vi "Benchmark VIReg(SubVI).vi"(11 "#Tags":i32) -> (0 "Values":dbl[](array[numeric]), 1 "Read Time":dbl, 2 "Write Time":dbl, 3 "Creation Time":dbl)   [LabVIEW 2019]
uses:
  <vilib>/GPower/VIRegister/Library/Typedefs/RegisterType.ctl
  <vilib>/GPower/VIRegister/Library/Convert/ToDBL.vi
  <vilib>/GPower/VIRegister/Library/QManager/CreateRegister.vi
  <vilib>/GPower/VIRegister/Library/SubVIs/FindRegisterData.vi
  <vilib>/GPower/VIRegister/Library/SubVIs/WriteSub.vi
  <vilib>/GPower/VIRegister/Library/SubVIs/ReadSub.vi
  <vilib>/GPower/Error/Library/IsError.vi
  <vilib>/GPower/VIRegister/Library/QManager/ReleaseAll.vi
  <vilib>/GPower/VIRegister/Library/QManager/QManagerAction.vi
  <vilib>/GPower/VIRegister/Library/QManager/GetRegisterData.vi
  <vilib>/GPower/Error/Library/SetError.vi
  <vilib>/GPower/Error/Library/FilterCodes.vi
  <vilib>/GPower/Error/Library/Filter/FilterMulti.vi
  <vilib>/GPower/Error/Library/ErrorType.vi
  <vilib>/GPower/Error/Library/SplitAppended.vi
  <vilib>/GPower/Error/Library/SubVIs/ExplanationToError.vi
  <vilib>/dlg_ctls.llb/Space Constant.vi
  <vilib>/GPower/VIRegister/Library/QManager/GetQName.vi
  <vilib>/GPower/VIRegister/Library/QManager/StartQManager.vi
  <vilib>/Utility/error.llb/Trim Whitespace.vi
  <vilib>/Utility/error.llb/Error Code Database.vi
  <vilib>/GPower/Error/Library/SubVIs/SetStatus.vi
  <vilib>/GPower/Error/Library/AppendErrors.vi
  <vilib>/GPower/Error/Library/Append/AppendSingle.vi
  <vilib>/GPower/VIRegister/VIRegister.lvlib
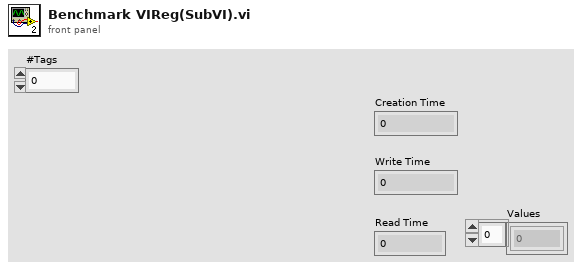
[diagram p1: front panel]
types:
  T1 = typedef "VIRegister.lvlib/RegisterType.ctl" = enum16{"Circular buffer", "FIFO buffer", "LIFO buffer", "Register"}
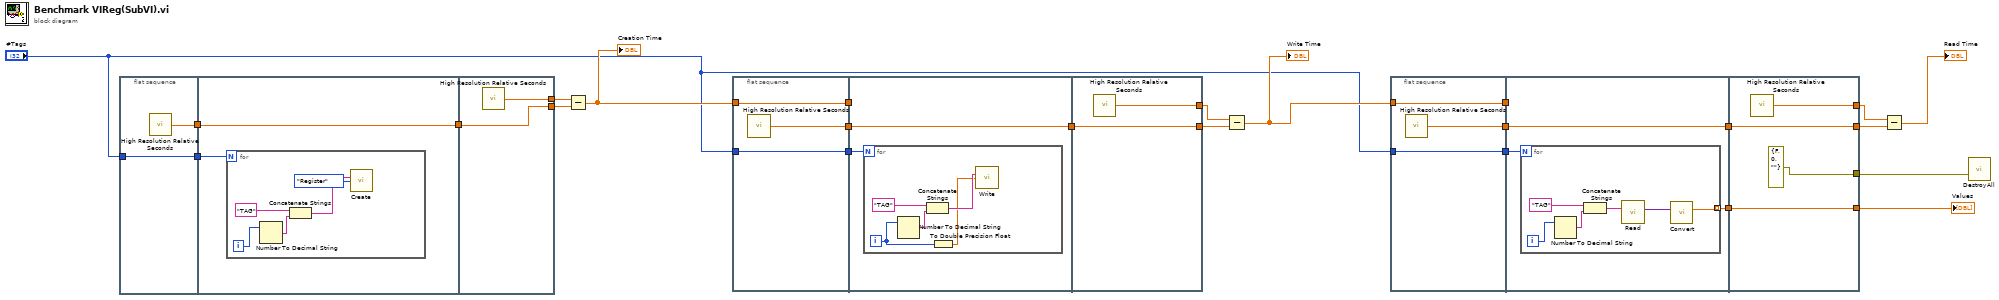
[diagram p0: block diagram]
diagram:
  n1 = flat-sequence {
    tunnel: "#Tags" -> [w26]
    tunnel: [w26] -> w24
    tunnel: [w25] -> w22
    tunnel: w24 -> [w28]
    tunnel: [w27] -> w23
    tunnel: w22 -> [w27]
    tunnel: w23 -> [w34]
    tunnel: [w35] -> w21
    tunnel: [w34] -> w20
    frame #0 {
      n2 = call <vilib>:"High Resolution Relative Seconds.vi"() -> ("relative seconds"=w25:dbl)
    }
    frame #1 {
      n3 = for {
        N: w28 -> [_]
        i -> [w32]
        n4 = Number To Decimal String(number=w32) -> (decimal integer string=w31:string)  [unwired: 1 in]
        n5 = Concatenate Strings("TAG", w31) -> (w30:string)
        n6 = call <vilib>:"Create.vi"("Register name"=w30, "Register type"=RegisterType."Register") -> ()  [unwired: 12 in, 2 out]
      }
    }
    frame #2 {
      n7 = call <vilib>:"High Resolution Relative Seconds.vi"() -> ("relative seconds"=w35:dbl)
    }
  }
  n8 = Subtract(x=w21, y=w20) -> (x-y=w19:dbl)
  "Creation Time" <- w19
  n9 = flat-sequence {
    tunnel: w19 -> [w38]
    tunnel: [w38] -> w18
    tunnel: [w37] -> w16
    tunnel: [w36] -> w15
    tunnel: "#Tags" -> [w36]
    tunnel: w18 -> [_]
    tunnel: [w40] -> w17
    tunnel: w16 -> [w40]
    tunnel: w15 -> [w39]
    tunnel: w17 -> [w47]
    tunnel: [w47] -> w13
    tunnel: [w46] -> w14
    frame #0 {
      n10 = call <vilib>:"High Resolution Relative Seconds.vi"() -> ("relative seconds"=w37:dbl)
    }
    frame #1 {
      n11 = for {
        N: w39 -> [_]
        i -> [w43]
        n12 = Number To Decimal String(number=w43) -> (decimal integer string=w44:string)  [unwired: 1 in]
        n13 = Concatenate Strings("TAG", w44) -> (w42:string)
        n14 = To Double Precision Float(number=w43) -> (double precision float=w41:dbl)
        n15 = call <vilib>:"Write.vi"("Register name"=w42, "Register value"=w41) -> ()  [unwired: 11 in, 3 out]
      }
    }
    frame #2 {
      n16 = call <vilib>:"High Resolution Relative Seconds.vi"() -> ("relative seconds"=w46:dbl)
    }
  }
  n17 = Subtract(x=w14, y=w13) -> (x-y=w5:dbl)
  "Write Time" <- w5
  n18 = flat-sequence {
    tunnel: w5 -> [w50]
    tunnel: [w50] -> w12
    tunnel: [w49] -> w11
    tunnel: [w48] -> w10
    tunnel: "#Tags" -> [w48]
    tunnel: w12 -> [_]
    tunnel: [w53] -> w9
    tunnel: w11 -> [w53]
    tunnel: w10 -> [w52]
    tunnel: [w51] -> w4
    tunnel: w9 -> [w63]
    tunnel: [w63] -> w7
    tunnel: [w62] -> w6
    tunnel: [w61] -> w3
    tunnel: w4 -> [w61]
    tunnel: [errorcluster {"status"=FALSE, "code"=0, "source"=""} ("error in (no error)")] -> w1
    frame #0 {
      n19 = call <vilib>:"High Resolution Relative Seconds.vi"() -> ("relative seconds"=w49:dbl)
    }
    frame #1 {
      n20 = for {
        N: w52 -> [_]
        tunnel: [w54] -> w51 mode=indexing
        i -> [w57]
        n21 = Number To Decimal String(number=w57) -> (decimal integer string=w58:string)  [unwired: 1 in]
        n22 = Concatenate Strings("TAG", w58) -> (w56:string)
        n23 = call <vilib>:"Read.vi"("Register name"=w56) -> ("Register value"=w55:variant)  [unwired: 11 in, 3 out]
        n24 = call-poly <vilib>:"Convert.vi"("Register value in"=w55) -> ("Register value out"=w54:dbl)  [unwired: 13 in, 1 out]
      }
    }
    frame #2 {
      n25 = call <vilib>:"High Resolution Relative Seconds.vi"() -> ("relative seconds"=w62:dbl)
    }
  }
  n26 = Subtract(x=w6, y=w7) -> (x-y=→"Read Time":dbl)
  n27 = call <vilib>:"DestroyAll.vi"("Error in"=w1) -> ()  [unwired: 13 in, 2 out]
  "Values" <- w3
